vi "thermo_init_retry.vi"(4 "error in (no error)":errorcluster, 5 "try fail in":T1(ring), 6 "retry N in":i32=-1, 7 "timeout in":i32=-1) -> (0 "error out":errorcluster, 1 "try fail out":T1(ring), 2 "retry N out":i32, 3 "timeout out":i32)   [LabVIEW 2020]
uses:
  thermo_var.vi
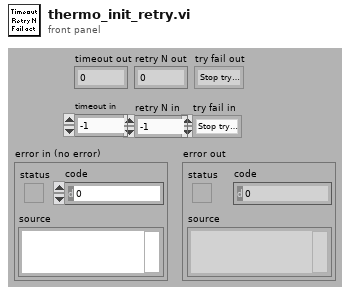
[diagram p1: front panel]
types:
  T1 = enum16{"Stop trying - keep last value", "Stop trying - return zeroes", "Generate error - stop sweep"}
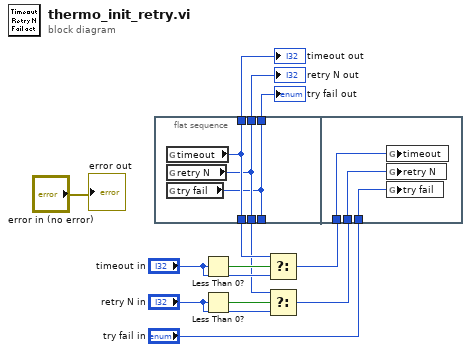
[diagram p0: block diagram]
diagram:
  n1 = flat-sequence {
    tunnel: [w16] -> w13
    tunnel: [w15] -> w12
    tunnel: [w14] -> w11
    tunnel: [w16] -> w8
    tunnel: [w15] -> w5
    tunnel: [w14] -> _
    tunnel: w4 -> [w19]
    tunnel: w3 -> [w18]
    tunnel: "try fail in" -> [w17]
    frame #0 {
      n2 = global read "thermo_var.vi" "timeout"() -> (w16:i32)
      n3 = global read "thermo_var.vi" "retry N"() -> (w15:i32)
      n4 = global read "thermo_var.vi" "try fail"() -> (w14:T1)
    }
    frame #1 {
      n5 = global write "thermo_var.vi" "timeout"(w19) -> ()
      n6 = global write "thermo_var.vi" "retry N"(w18) -> ()
      n7 = global write "thermo_var.vi" "try fail"(w17) -> ()
    }
  }
  n8 = Less Than 0?(x="timeout in") -> (x < 0?=w10:bool)
  n9 = Less Than 0?(x="retry N in") -> (x < 0?=w7:bool)
  n10 = Select(t=w8, s=w10, f="timeout in") -> (s? t:f=w4:i32)
  n11 = Select(t=w5, s=w7, f="retry N in") -> (s? t:f=w3:i32)
  "timeout out" <- w13
  "retry N out" <- w12
  "try fail out" <- w11
  "error out" <- "error in (no error)"
